vi "Read.vi"(7 "length":u16, 8 "error in (no error)":errorcluster, 9 "Start address":string, 10 "Read Type":variant, 11 "MelsecTCP in":refnum<class "Abstract PLC Controler.lvclass">) -> (0 "error out":errorcluster, 2 "Data":variant, 3 "MelsecTCP out":refnum<class "Abstract PLC Controler.lvclass">)   [LabVIEW 2020, in "HslCommunication.lvlib" / "Abstract PLC Controler.lvclass"]
uses:
  Abstract PLC Controler.lvclass
  EventLogger.lvlibp/1abvi3w/vi.lib/gpm_packages/@cs/event-logger/Source/Composed Log/Types/Log Level.ctl
  Abstract PLC Controler.lvclass/Abstract PLC Controler.ctl
  EventLogger.lvlibp/1abvi3w/vi.lib/gpm_packages/@cs/event-logger/Source/Composed Log/Composed Log.lvlib
  EventLogger.lvlibp/Logger.lvclass
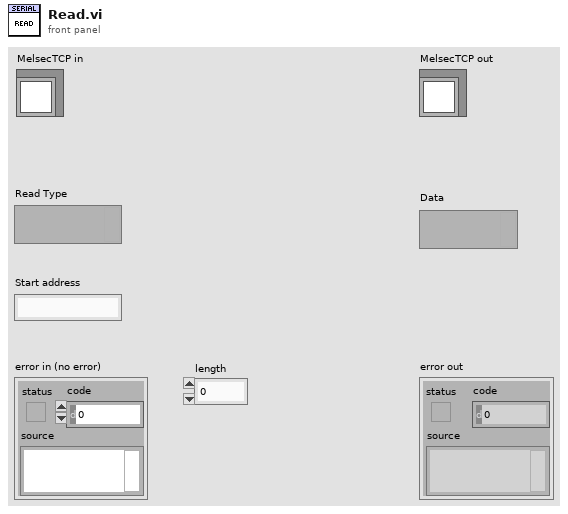
[diagram p1: front panel]
types:
  T1 = typedef "EventLogger.lvlibp/Composed Log.lvlib/Log Level.ctl" = enum16{"Debug", "Info", "Warning", "Error", "Critical"}
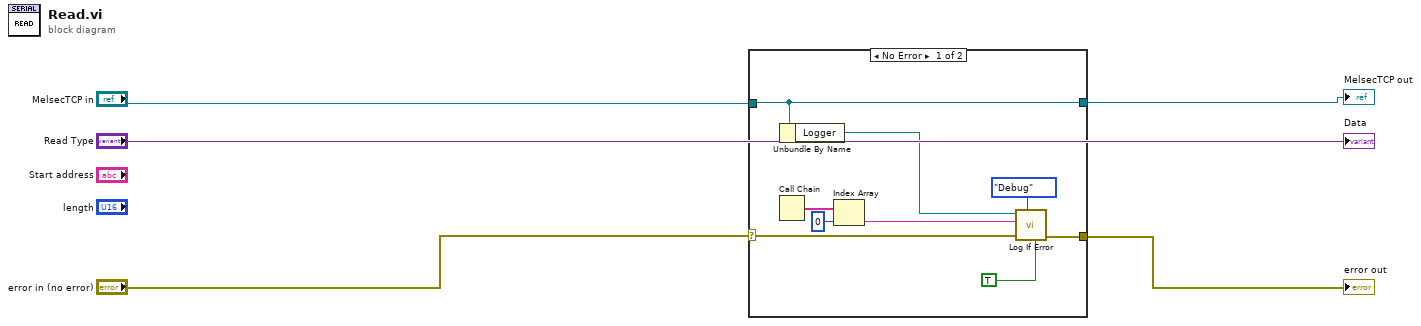
[diagram p0: block diagram]
diagram:
  n1 = case shown="No Error" "error in (no error)" {
    selector: "error in (no error)" -> [w14 w16]
    tunnel: [w13 w16] -> w3
    tunnel: "MelsecTCP in" -> [w6 w15]
    tunnel: [w6 w15] -> w4
    frame No Error {
      n2 = Call Chain() -> (call chain=w10:string[])
      n3 = Unbundle By Name(w6) -> ("Logger"=w12:refnum<class "Logger.lvclass">)
      n4 = Index Array(array=w10, index=0) -> (element=w8:string)
      n5 = call "Log If Error.vi"("Include Warnings(F)"=TRUE, "Event Level (Error)"=Log_Level."Debug", "error in (no error)"=w14, "SourceID"=w8, "Logger in"=w12) -> ("error out"=w13:errorcluster)  [unwired: 5 in, 1 out]
    }
    frame Error {
    }
  }
  "error out" <- w3
  "MelsecTCP out" <- w4
  "Data" <- "Read Type"
